vi "Scale.vi"(8 "error in (no error)":errorcluster, 10 "Scale Factor":dbl, 11 "Line in":refnum<class "Line.lvclass">) -> (0 "error out":errorcluster, 3 "Line out":refnum<class "Line.lvclass">)   [LabVIEW 2021, in "Picture2D.lvlib" / "Line.lvclass"]
uses:
  Line.lvclass
  Shape/Shape.lvclass
  Point/Point.lvclass
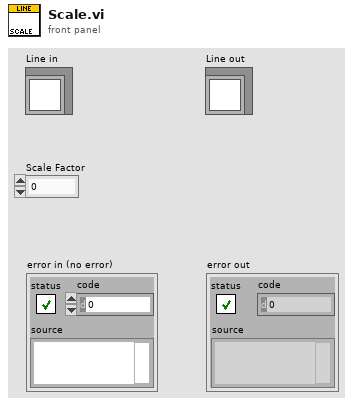
[diagram p1: front panel]
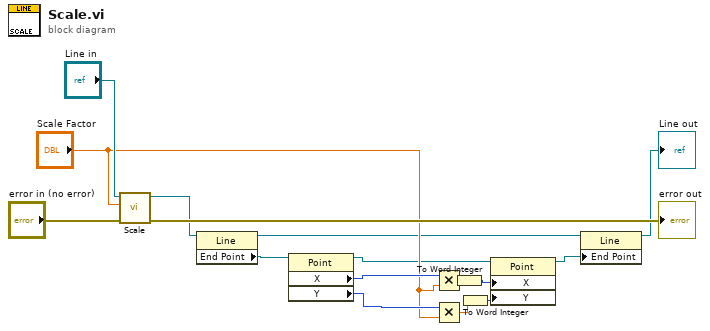
[diagram p0: block diagram]
diagram:
  n1 = call-parent "Scale.vi"("error in (no error)"="error in (no error)", "Scale Factor"="Scale Factor", "Shape in"="Line in") -> ("error out"=→"error out":errorcluster, "Shape out"=w13:refnum<class "Line.lvclass">)  [unwired: 7 in]
  n2 = property class="Line"(reference=w13) -> (reference out=w2:refnum<class "Line.lvclass">, "End Point"=w11:refnum<class "Point.lvclass">)  [unwired: 1 in, 1 out]
  n3 = property class="Point"(reference=w11) -> (reference out=w1:refnum<class "Point.lvclass">, "X"=w10:i16, "Y"=w9:i16)  [unwired: 1 in, 1 out]
  n4 = Multiply(x=w10, y="Scale Factor") -> (x*y=w6:dbl)
  n5 = Multiply(x=w9, y="Scale Factor") -> (x*y=w5:dbl)
  n6 = To Word Integer(number=w6) -> (16bit integer=w4:i16)
  n7 = To Word Integer(number=w5) -> (16bit integer=w3:i16)
  n8 = property class="Point"(reference=w1, "X"=w4, "Y"=w3) -> (reference out=w7:refnum<class "Point.lvclass">)  [unwired: 1 in, 1 out]
  n9 = property class="Line"(reference=w2, "End Point"=w7) -> (reference out=→"Line out":refnum<class "Line.lvclass">)  [unwired: 1 in, 1 out]
